vi "sendValue.vi"(8 "error in (no error)":errorcluster, 10 "data":variant, 11 "setMode in":refnum<class "setMode.lvclass">) -> (0 "error out":errorcluster, 2 "function return":i32, 3 "setMode out":refnum<class "setMode.lvclass">)   [LabVIEW 2016, in "SALLV_MtAtElectrometer_Messaging.lvlib" / "setMode.lvclass"]
uses:
  setMode.lvclass
  ts_sallv_MtAtElectrometer/DataTypes/command_setMode.ctl
  ts_sallv_MtAtElectrometer/SALLV_MtAtElectrometer.lvlib
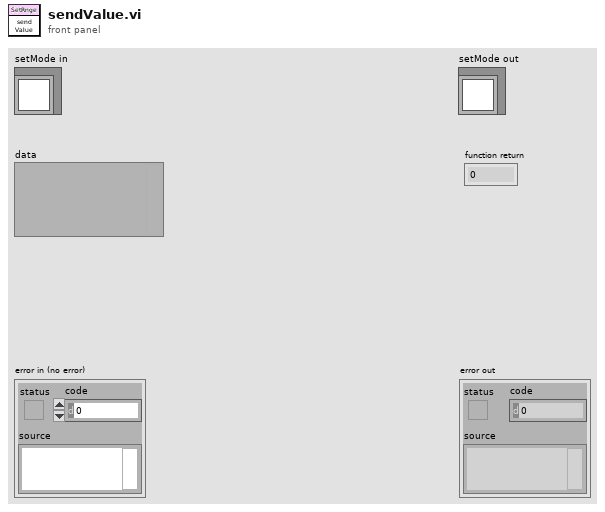
[diagram p1: front panel]
types:
  T1 = typedef "SALLV_MtAtElectrometer.lvlib/command_setMode.ctl" = cluster{"mode":u16}
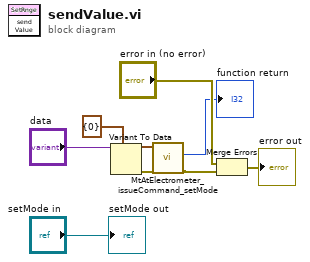
[diagram p0: block diagram]
diagram:
  n1 = Variant To Data(type=T1 {"mode"=0} ("command_setMode_Ctl"), Variant="data") -> (data=w3:T1, error out=w5:errorcluster)  [unwired: 1 in]
  n2 = call "MtAtElectrometer_issueCommand_setMode.vi"("error in (no error)"=w5, "command_setMode_Ctl"=w3) -> ("error out"=w4:errorcluster, "function return"=→"function return":i32)  [unwired: 7 in, 1 out]
  n3 = Merge Errors("error in (no error)", w4) -> (→"error out":errorcluster)
  "setMode out" <- "setMode in"
